vi "CheckCurrentStatus.vi"() -> (2 "body":string, 3 "headers":string)   [LabVIEW 2020]
uses:
  <vilib>/httpClient/LabVIEWHTTPClient.lvlib
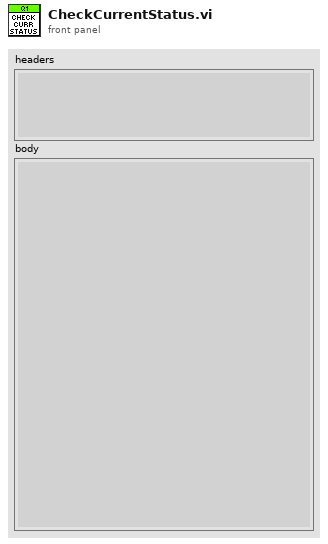
[diagram p1: front panel]
types:
  T1 = typedef "LabVIEWHTTPClient.lvlib/ClientHandle.ctl" = refnum<k1>
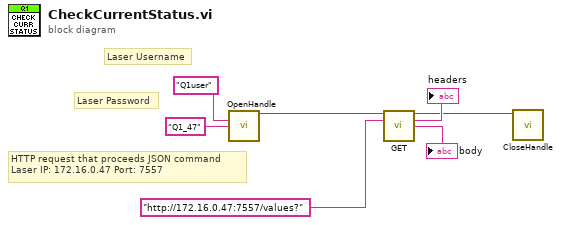
[diagram p0: block diagram]
diagram:
  # "HTTP request that proceeds JSON command\nLaser IP: 172.16.0.47 Port: 7557"
  # "Laser Password"
  # "Laser Username"
  n1 = call <vilib>:"OpenHandle.vi"("username"="Q1user", "password"="Q1_47") -> ("client handle out"=w5:T1)  [unwired: 12 in, 1 out]
  n2 = call <vilib>:"GET.vi"("client handle"=w5, "url"="http://172.16.0.47:7557/values?") -> ("client handle out"=w2:T1, "headers"=→"headers":string, "body"=→"body":string)  [unwired: 10 in, 1 out]
  n3 = call <vilib>:"CloseHandle.vi"("client handle"=w2) -> ()  [unwired: 14 in, 1 out]
